vi "Set Object Item by name.vi"(8 "error in (no error)":errorcluster, 9 "name":string, 10 "Value":refnum<class "JSON Value.lvclass">, 11 "JSON Object in":refnum<class "JSON Object.lvclass">) -> (0 "error out":errorcluster, 1 "replaced":bool, 3 "JSON Object out":refnum<class "JSON Object.lvclass">)   [LabVIEW 2020, in "Library Commun.lvlib" / "JSON Object.lvclass"]
doc: "Stores a <b>JSON Value</b> in a <b>JSON Object</b> by it's name.\n\nCopyright 2012 James David Powell, Shaun Rumbell and Ton Plomp\nMore information on http://lavag.org/topic/16217-cr-json-labview"
uses:
  JSON Object.lvclass
  JSON Value/JSON Value.lvclass
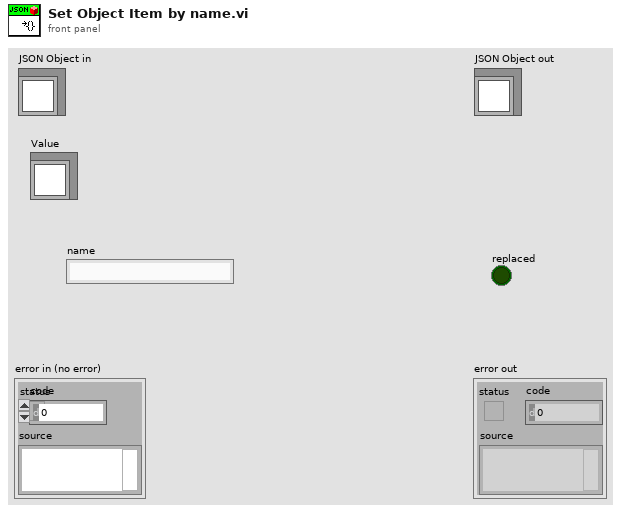
[diagram p1: front panel]
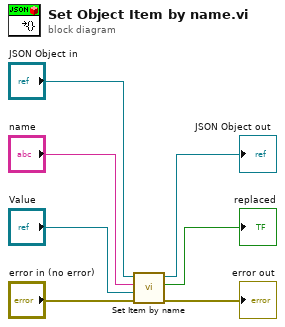
[diagram p0: block diagram]
diagram:
  n1 = call-dynamic "Set Item by name.vi"("error in (no error)"="error in (no error)", "Value"="Value", "name"="name", "JSON Object in"="JSON Object in") -> ("error out"=→"error out":errorcluster, "replaced"=→"replaced":bool, "JSON Object out"=→"JSON Object out":refnum<class "JSON Object.lvclass">)  [unwired: 5 in]
